vi "Actor Core.vi"(8 "error in":errorcluster, 11 "ES in":refnum<class "ES.lvclass">) -> (0 "error out":errorcluster, 3 "Actor out":refnum<class "Actor.lvclass">)   [LabVIEW 2018, in "ES Actor.lvlib" / "ES.lvclass"]
doc: "(<B>Filename</B>: Actor Framework.lvlib:Actor.lvclass:Actor Core.vi)\n\nReceives messages to the actor, reacts to them, and initiates any error handling that may shut the actor down.\n\nDescendant classes may override this VI to append parallel tasks for the actor to complete while it handles messages. Overrides use the Call Parent Method node."
uses:
  ES.lvclass
  C:/Users/Administrator/Desktop/2018LabVIEW EMS/EMS Generic Actor/EMS Generic/EMS Generic.lvclass
  <vilib>/ActorFramework/Actor/Actor.lvclass
  EMS Generic Actor/EMS Generic/EMS Generic.lvclass/EMS Generic.ctl
  <vilib>/ORNL/CSEISMIC DDS/CSEISMIC DDS Base/CSEISMIC DDS.lvclass/CSEISMIC DDS.ctl
  <vilib>/ORNL/CSEISMIC DDS/CSEISMIC DDS Base/Accessors/Write DDS Reference.vi
  <vilib>/ORNL/CSEISMIC DDS/CSEISMIC DDS Base/Accessors/Read DDS Reference.vi
  <vilib>/ORNL/CSEISMIC DDS/DDS Reader/DDS Reader.lvclass
  C:/Program Files (x86)/National Instruments/LabVIEW 2018/vi.lib/ORNL/CSEISMIC DDS/CSEISMIC DDS Base/CSEISMIC DDS.lvclass
  <vilib>/ORNL/CSEISMIC DDS/CSEISMIC DDS Base/Error Handler.vi
  Device DDS Communications Framework/Device DDS Communications/Device DDS Communications.lvclass
  EMS Generic Actor/EMS Generic/EMS Generic.lvclass
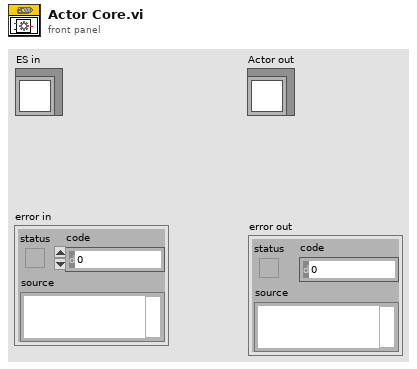
[diagram p1: front panel]
types:
  T1 = typedef "CSEISMIC DDS.lvlib/CSEISMIC DDS.lvclass/DeviceID.ctl" = string
  T2 = typedef "CSEISMIC DDS.lvlib/CSEISMIC DDS.lvclass/ES_Info.ctl" = cluster{"DeviceID":T1, "EnergyRating (kWh)":dbl, "RampRate (kW/s)":dbl, "MaxPowerFactorLeading":dbl, "MaxPowerFactorLagging":dbl, "ChargingEfficiencyCurve":T3, "DischargingEfficiencyCurve":T3, "MinSOC (%)":dbl, "MaxSOC (%)":dbl}
  T3 = typedef "CSEISMIC DDS.lvlib/CSEISMIC DDS.lvclass/EfficiencyCurve.ctl" = cluster{"Power (kW)":dbl[], "Efficiency (%)":dbl[]}
  T4 = typedef "LVDDS_library.lvlib/DDS Sample Info.ctl" = cluster{"DDS_SampleStateKind":enum32{"DDS_INVALID_SAMPLE_STATE", "DDS_READ_SAMPLE_STATE", "DDS_NOT_READ_SAMPLE_STATE"}, "DDS_ViewStateKind":enum32{"DDS_INVALID_SAMPLE_STATE", "DDS_NEW_VIEW_STATE", "DDS_NOT_NEW_VIEW_STATE"}, "DDS_InstanceStateKind":enum32{"DDS_INVALID_STATE", "DDS_ALIVE_INSTANCE_STATE", "DDS_NOT_ALIVE_DISPOSED_INSTANCE_STATE", "", "DDS_NOT_ALIVE_NO_WRITERS_INSTANCE_STATE"}, "sec":i32, "nanosec":u32, "valid_data":bool}
  T5 = typedef "CSEISMIC DDS.lvlib/CSEISMIC DDS.lvclass/ES_Measurement.ctl" = cluster{"DeviceID":T1, "SOC (%)":dbl}
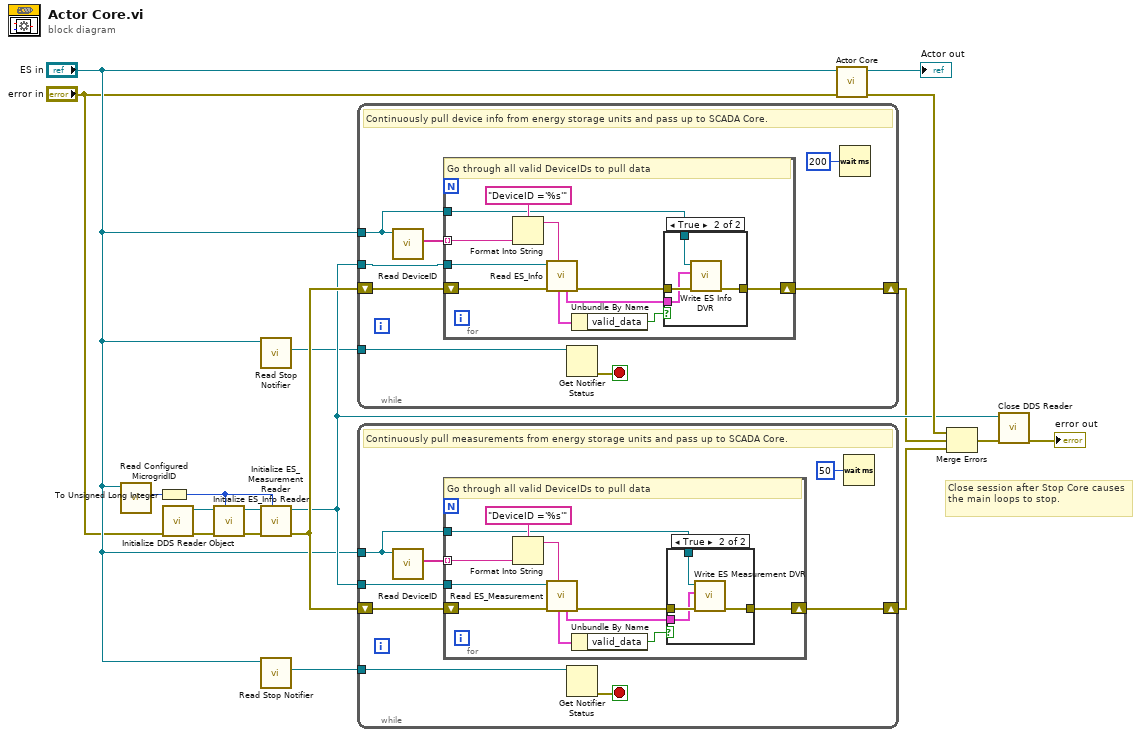
[diagram p0: block diagram]
diagram:
  # "Close session after Stop Core causes the main loops to stop."
  n1 = call "Read Configured MicrogridID.vi"("EMS Generic in"="ES in") -> ("Microgrid ID"=w18:u8)  [unwired: 8 in, 2 out]
  n2 = To Unsigned Long Integer(number=w18) -> (unsigned 32bit integer=w3:u32)
  n3 = call <vilib>:"Initialize DDS Reader Object.vi"("error in"="error in") -> ("error out"=w14:errorcluster, "DDS Reader out"=w13:refnum<class "DDS Reader.lvclass">)  [unwired: 9 in]
  n4 = call <vilib>:"Initialize ES_Info Reader.vi"("MicrogridID"=w3, "error in"=w14, "DDS Reader in"=w13) -> ("error out"=w15:errorcluster, "DDS Reader out"=w12:refnum<class "DDS Reader.lvclass">)  [unwired: 7 in]
  n5 = call "Read Stop Notifier.vi"("EMS Generic in"="ES in") -> ("stop"=w6:refnum<notifier>)  [unwired: 9 in, 1 out]
  n6 = call <vilib>:"Initialize ES_Measurement Reader.vi"("MicrogridID"=w3, "error in"=w15, "DDS Reader in"=w12) -> ("error out"=w11:errorcluster, "DDS Reader out"=w10:refnum<class "DDS Reader.lvclass">)  [unwired: 7 in]
  n7 = call "Read Stop Notifier.vi"("EMS Generic in"="ES in") -> ("stop"=w5:refnum<notifier>)  [unwired: 9 in, 1 out]
  n8 = while {
    tunnel: w6 -> [w26]
    shift-right: [w19] -> w9
    shift-left: w11 -> [w22]
    tunnel: "ES in" -> [w20]
    tunnel: w10 -> [w21]
    stop <- w25 stop-if-true
    # "Continuously pull device info from energy storage units and pass up to SCADA Core."
    n9 = call-dynamic "Read DeviceID.vi"("Device DDS Communications in"=w20) -> ("DeviceID"=w23:T1[])  [unwired: 9 in, 1 out]
    n10 = for {
      shift-right: [w28] -> w19
      shift-left: w22 -> [w36]
      tunnel: w23 -> [w34] mode=indexing
      tunnel: w21 -> [w37]
      tunnel: w20 -> [w27]
      # "Go through all valid DeviceIDs to pull data"
      n11 = Format Into String(format string="DeviceID ='%s'", w34) -> (resulting string=w33:string)  [unwired: 2 in, 1 out]
      n12 = call <vilib>:"Read ES_Info.vi"("Query condition"=w33, "error in"=w36, "DDS Reader in"=w37) -> ("error out"=w29:errorcluster, "data"=w30:T2, "DDS Sample Info"=w32:T4)  [unwired: 5 in, 1 out]
      n13 = Unbundle By Name(w32) -> ("valid_data"=w31:bool)
      n14 = case shown="True" w31 {
        tunnel: w30 -> [_ w40]
        tunnel: w29 -> [w38 w42]
        tunnel: [w38 w41] -> w28
        tunnel: w27 -> [_ w39]
        frame False {
        }
        frame True {
          n15 = call "Write ES Info DVR.vi"("error in"=w42, "ES_Info"=w40, "EMS Generic in"=w39) -> ("error out"=w41:errorcluster)  [unwired: 7 in, 1 out]
        }
      }
    }
    n16 = Get Notifier Status(notifier=w26) -> (error out=w25:errorcluster)  [unwired: 1 in, 4 out]
    n17 = Wait (ms)(milliseconds to wait=u32 200) -> ()  [unwired: 1 out]
  }
  n18 = while {
    tunnel: w5 -> [w50]
    shift-right: [w44] -> w8
    shift-left: w11 -> [w46]
    tunnel: "ES in" -> [w43]
    tunnel: w10 -> [w45]
    stop <- w49 stop-if-true
    # "Continuously pull measurements from energy storage units and pass up to SCADA Core."
    n19 = call-dynamic "Read DeviceID.vi"("Device DDS Communications in"=w43) -> ("DeviceID"=w47:T1[])  [unwired: 9 in, 1 out]
    n20 = for {
      shift-right: [w52] -> w44
      shift-left: w46 -> [w60]
      tunnel: w47 -> [w58] mode=indexing
      tunnel: w45 -> [w61]
      tunnel: w43 -> [w51]
      # "Go through all valid DeviceIDs to pull data"
      n21 = Format Into String(format string="DeviceID ='%s'", w58) -> (resulting string=w57:string)  [unwired: 2 in, 1 out]
      n22 = call <vilib>:"Read ES_Measurement.vi"("Query condition"=w57, "error in"=w60, "DDS Reader in"=w61) -> ("error out"=w53:errorcluster, "data"=w54:T5, "DDS Sample Info"=w56:T4)  [unwired: 5 in, 1 out]
      n23 = Unbundle By Name(w56) -> ("valid_data"=w55:bool)
      n24 = case shown="True" w55 {
        tunnel: w54 -> [_ w64]
        tunnel: w53 -> [w62 w66]
        tunnel: [w62 w65] -> w52
        tunnel: w51 -> [_ w63]
        frame False {
        }
        frame True {
          n25 = call "Write ES Measurement DVR.vi"("error in"=w66, "ES_Measurement"=w64, "EMS Generic in"=w63) -> ("error out"=w65:errorcluster)  [unwired: 7 in, 1 out]
        }
      }
    }
    n26 = Get Notifier Status(notifier=w50) -> (error out=w49:errorcluster)  [unwired: 1 in, 4 out]
    n27 = Wait (ms)(milliseconds to wait=u32 50) -> ()  [unwired: 1 out]
  }
  n28 = call-parent "Actor Core.vi"("error in"="error in", "Actor in"="ES in") -> ("error out"=w16:errorcluster, "Actor out"=→"Actor out":refnum<class "Actor.lvclass">)  [unwired: 8 in]
  n29 = Merge Errors(w16, w9, w8) -> (w7:errorcluster)
  n30 = call <vilib>:"Close DDS Reader.vi"("error in"=w7, "DDS Reader in"=w10) -> ("error out"=→"error out":errorcluster)  [unwired: 9 in]
